vi "Read Write ADS State.vi"() -> ()   [LabVIEW 2018]
uses:
  TwinCAT ADS Class/Controls/State Information.ctl
  TwinCAT ADS Class/TwinCAT ADS.lvclass
panel:
  in  "Read/Write":enum16{"Read State", "Write ADS State"}(ring)
  in  "ADS State":i16(ring) items=["Invalid", "Idle", "Reset", "Init", "Start", "Run", "Stop", "SaveConfig", "LoadConfig", "PowerFailure", "PowerGood", "Error", "Shutdown", "Suspend", "Resume", "Config", "Reconfig", "Stopping, Maxstates", "Incompatible", "Exception"]
  out "State Information":T1
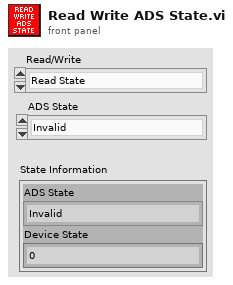
[diagram p1: front panel]
types:
  T1 = typedef "TwinCAT ADS.lvclass/State Information.ctl" = cluster{"ADS State":enum16{"Invalid", "Idle", "Reset", "Init", "Start", "Run", "Stop", "SaveConfig", "LoadConfig", "PowerFailure", "PowerGood", "Error", "Shutdown", "Suspend", "Resume", "Config", "Reconfig", "Stopping, Maxstates", "Incompatible", "Exception"}, "Device State":i16}
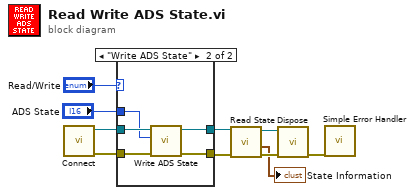
[diagram p0: block diagram]
diagram:
  n1 = call "Connect.vi"() -> ("error out"=w9:errorcluster, "TwinCAT ADS out"=w8:refnum<class "TwinCAT ADS.lvclass">)  [unwired: 10 in]
  n2 = case shown="\"Write ADS State\"" "Read/Write" {
    tunnel: w9 -> [w11 w17]
    tunnel: w8 -> [w12 w16]
    tunnel: "ADS State" -> [_ w15]
    tunnel: [w12 w14] -> w6
    tunnel: [w11 w13] -> w5
    frame "Read State", Default {
    }
    frame "Write ADS State" {
      n3 = call "Write ADS State.vi"("error in (no error)"=w17, "ADS State"=w15, "TwinCAT ADS in"=w16) -> ("error out"=w13:errorcluster, "TwinCAT ADS out"=w14:refnum<class "TwinCAT ADS.lvclass">)  [unwired: 7 in]
    }
  }
  n4 = call "Read State.vi"("error in (no error)"=w5, "TwinCAT ADS in"=w6) -> ("error out"=w3:errorcluster, "State Information"=→"State Information":T1, "TwinCAT ADS out"=w4:refnum<class "TwinCAT ADS.lvclass">)  [unwired: 7 in]
  n5 = call "Dispose.vi"("error in (no error)"=w3, "TwinCAT ADS in"=w4) -> ("error out"=w1:errorcluster)  [unwired: 9 in]
  n6 = call <vilib>:"Simple Error Handler.vi"("error in (no error)"=w1) -> ()  [unwired: 4 in, 5 out]
